vi "Create ObjectBuffer.vi"(6 "buffer-type":T1, 7 "Allow Overflow? (T)":bool=TRUE, 8 "error in":errorcluster, 10 "default":refnum<class>, 11 "bufSize":i32) -> (0 "error out":errorcluster, 3 "Buffer":refnum<data-value>)   [LabVIEW 2013, in "CircularBuffer.lvlib" / "ObjectBuffer.lvclass"]
doc: "This VI creates a ring buffer of set size. This buffer is created in one place in the memory and is then accessed via pointer/reference.\n\nThe Data Type input is required because it defines the place in the memory to correct size thus removing the need for memory reallocation."
uses:
  ObjectBuffer.lvclass
  VariantBuffer/buffer-type -- enum.ctl
  VariantBuffer/VariantBuffer.lvclass
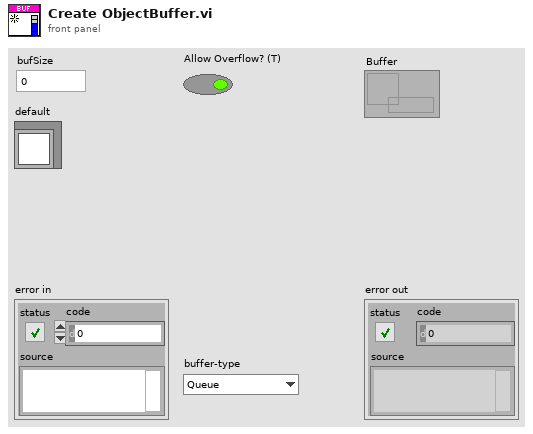
[diagram p1: front panel]
types:
  T1 = typedef "CircularBuffer.lvlib/VariantBuffer.lvclass/buffer-type -- enum.ctl" = enum16{"Queue", "Stack"}
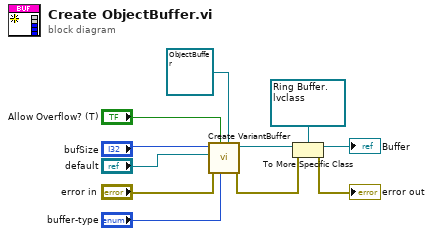
[diagram p0: block diagram]
diagram:
  n1 = call "Create VariantBuffer.vi"("Buffer"=refnum<class "ObjectBuffer.lvclass"> refnum ("Ring Buffer.lvclass"), "buffer-type"="buffer-type", "Allow Overflow? (T)"="Allow Overflow? (T)", "error in"="error in", "default"="default", "bufSize"="bufSize") -> ("error out"=w3:errorcluster, "Buffer"=w10:refnum<data-value>)  [unwired: 4 in]
  n2 = To More Specific Class(target class=refnum<data-value> refnum ("Buffer"), reference=w10, error in=w3) -> (specific class reference=→"Buffer":refnum<data-value>, error out=→"error out":errorcluster)
